vi "TriggerRefresh.vi"(0 "TriggerSetting引用句柄":refnum<vi>) -> ()   [LabVIEW 2012]
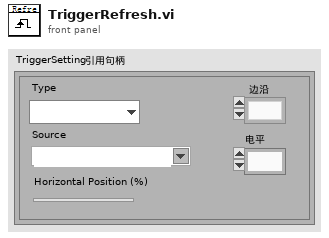
[diagram p1: front panel]
types:
  T1 = enum8{"Enabled", "Disabled", "Disabled and Grayed Out"}
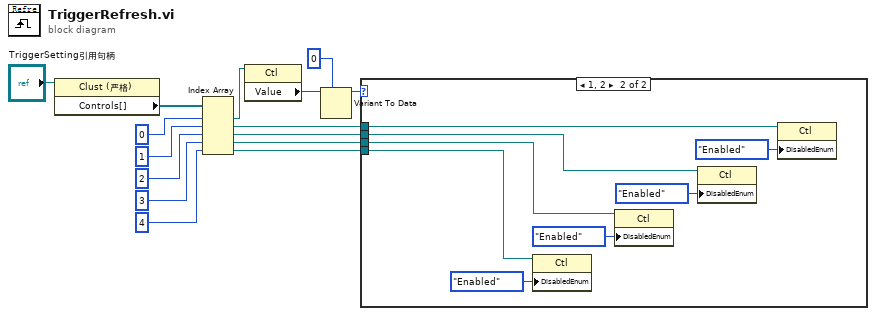
[diagram p0: block diagram]
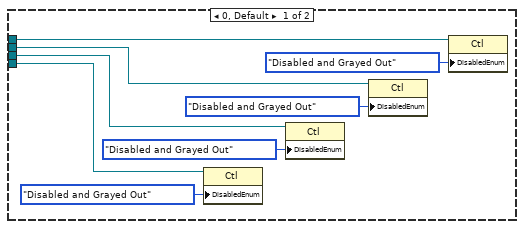
[diagram p2: hidden frame]
diagram:
  n1 = property class="Clust (严格)"(reference="TriggerSetting引用句柄") -> ("Controls[]"=w14:refnum<vi>[])  [unwired: 1 in, 2 out]
  n2 = Index Array(array=w14, index #1=0 ("索引"), index #2=1 ("索引"), index #3=2 ("索引"), index #4=3 ("索引"), index #5=4 ("索引")) -> (element #1=w12:refnum<vi>, element #2=w4:refnum<vi>, element #3=w3:refnum<vi>, element #4=w2:refnum<vi>, element #5=w1:refnum<vi>)
  n3 = property class="Ctl"(reference=w12) -> ("Value"=w11:variant)  [unwired: 1 in, 2 out]
  n4 = Variant To Data(type=0, Variant=w11) -> (data=w9:i32)  [unwired: 1 in, 1 out]
  n5 = case shown="1, 2" w9 {
    tunnel: w4 -> [w19 w28]
    tunnel: w3 -> [w18 w25]
    tunnel: w2 -> [w17 w26]
    tunnel: w1 -> [w16 w27]
    frame 0, Default {
      n6 = property class="Ctl"(reference=w16, "DisabledEnum"=T1."Disabled and Grayed Out" ("禁用")) -> ()  [unwired: 1 in, 2 out]
      n7 = property class="Ctl"(reference=w17, "DisabledEnum"=T1."Disabled and Grayed Out" ("禁用")) -> ()  [unwired: 1 in, 2 out]
      n8 = property class="Ctl"(reference=w18, "DisabledEnum"=T1."Disabled and Grayed Out" ("禁用")) -> ()  [unwired: 1 in, 2 out]
      n9 = property class="Ctl"(reference=w19, "DisabledEnum"=T1."Disabled and Grayed Out" ("禁用")) -> ()  [unwired: 1 in, 2 out]
    }
    frame 1, 2 {
      n10 = property class="Ctl"(reference=w27, "DisabledEnum"=T1."Enabled" ("禁用")) -> ()  [unwired: 1 in, 2 out]
      n11 = property class="Ctl"(reference=w26, "DisabledEnum"=T1."Enabled" ("禁用")) -> ()  [unwired: 1 in, 2 out]
      n12 = property class="Ctl"(reference=w25, "DisabledEnum"=T1."Enabled" ("禁用")) -> ()  [unwired: 1 in, 2 out]
      n13 = property class="Ctl"(reference=w28, "DisabledEnum"=T1."Enabled" ("禁用")) -> ()  [unwired: 1 in, 2 out]
    }
  }
